vi "Puls Loop.vi"(1 "Loop ID":u16, 11 "error out":errorcluster) -> ()   [LabVIEW 2011]
uses:
  Update frequensies.ctl
  Action Analog Handler.ctl
  emi Lib/System 01/0 - General/App/Loop control 2/Private/_emi_ SMLoop start condition.vi
  emi Lib/System 01/0 - General/App/Loop control 2/Private/_emi_ SMLoop Error Check.vi
  emi Lib/Basic/0 - General/Error/emi_Is Error.vi
  emi Lib/System 01/0 - General/App/Loop control 2/Private/_emi_SMLoop Register new.vi
  emi Lib/System 01/0 - General/S&E reporting/emi_Send S&E Error message.vi
  emi Lib/Basic/0 - General/Error/emi_ Is Error state.vi
  emi Lib/System 01/0 - General/emi_Read System ID.vi
  emi Lib/System 01/0 - General/App/Loop control/Private/_emi_GFV Loop Linking.vi
  emi Lib/System 01/0 - General/App/Loop control/Private/_emi_GFV Loop Enable.vi
  emi Lib/System 01/0 - General/App/Loop control 2/Private/_emi_ SMLoop Restart.vi
  emi Lib/System 01/0 - General/App/Private/_emi_GFV App Close.vi
  emi Lib/System 01/0 - General/App/Loop control 2/Private/_emi_ SMLoop Restart Counter.vi
  emi Lib/System 01/0 - General/App/Loop control/Private/_emi_GFV Loop Running.vi
  emi Lib/System 01/0 - General/Private/_emi_GFV System ID.vi
  emi Lib/System 01/0 - General/S&E reporting/Private/_emi_S&E Q Generator.vi
  <vilib>/Utility/error.llb/Clear Errors.vi
  emi Lib/System 01/0 - General/App/Loop control/Private/_emi_GFV stop a loop so it can reset.vi
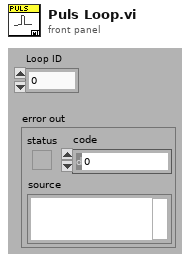
[diagram p1: front panel]
types:
  T1 = typedef "_emi_ SMLoop sates.ctl" = enum16{"Init", "Standby", "Start", "Normal Operation", "Stop", "Error Handling", "End", "Post"}
  T2 = typedef "Update frequensies.ctl" = enum16{"2 Hz", "1 Hz", "0.1 Hz"}
  T3 = typedef "Action Analog Handler.ctl" = enum16{"GET value", "GET Single Frequenzy", "GET All Values", "GET Waveform", "Get Numb Var", "SET Value", "START Buffer", "REG Variable", "BUF size(total antal sekund)", "PULS", "Get a Value at time", "Set initial waveform"}
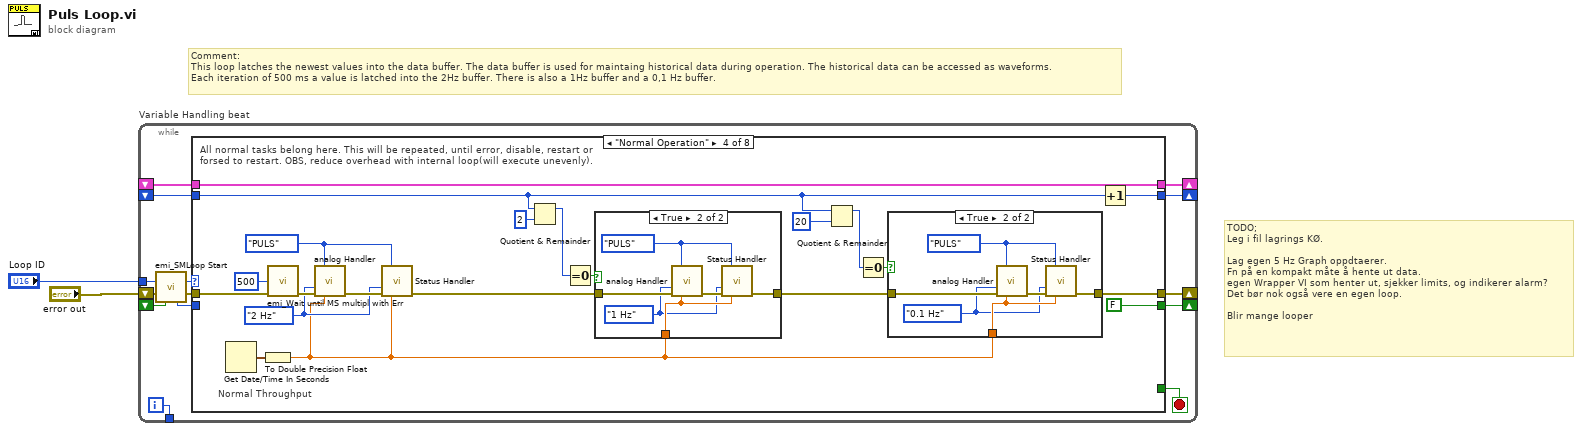
[diagram p0: block diagram]
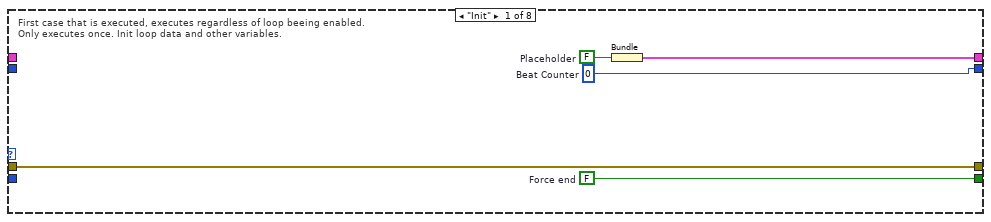
[diagram p2: hidden frame]
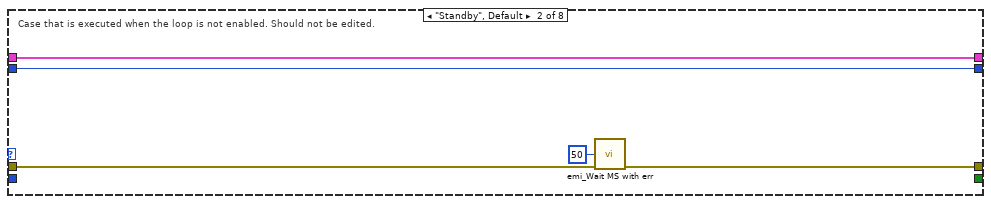
[diagram p3: hidden frame]
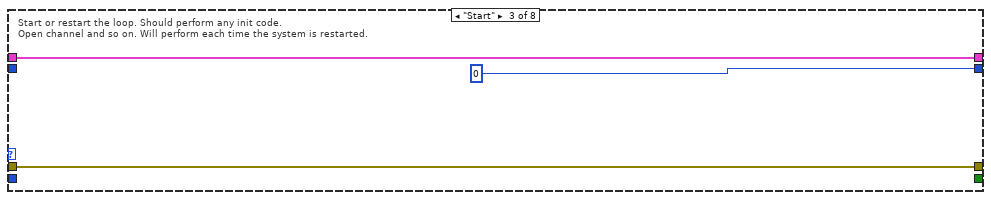
[diagram p4: hidden frame]
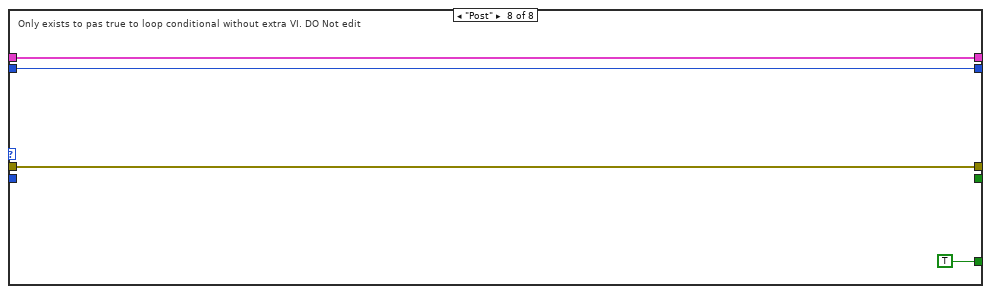
[diagram p10: hidden frame]
diagram:
  # "Comment: \nThis loop latches the newest values into the data buffer. The data buffer is used for maintaing historical data during operation. The historical data can be accessed as waveforms.\nEach iteration of 500 ms a value is latched into the 2Hz buffer. There is also a 1Hz buffer and a 0,1 Hz buffer."
  # "TODO;\nLeg i fil lagrings KØ.\n\nLag egen 5 Hz Graph oppdtaerer.\nFn på en kompakt måte å hente ut data.\negen Wrapper VI som henter ut, sjekker limits, og indikerer alarm?\nDet bør nok også vere en egen loop.\n\nBlir mange looper"
  n1 = while "Variable Handling beat" {
    shift-right: [w16] -> _
    shift-left: _ -> [w12]
    shift-right: [w14] -> _
    shift-left: "error out" -> [w10]
    tunnel: [w13] -> _
    shift-right: [w11] -> _
    shift-left: _ -> [w6]
    tunnel: "Loop ID" -> [w7]
    shift-right: [w3] -> _
    shift-left: _ -> [w4]
    i -> [w13]
    stop <- w15 stop-if-true
    n2 = call "emi_SMLoop Start.vi"("Loop ID"=w7, "error in (no error)"=w10, "Force Stop(F)"=w6) -> ("Loop command"=w8:T1, "error out"=w9:errorcluster, "Loop ID out"=w5:i32)  [unwired: 10 in]
    n3 = case shown="\"Normal Operation\"" w8 {
      tunnel: [w20 w23 w28 w48 w66 w70 w72 w76] -> w16
      tunnel: [_ _ _ _ _ _ _ TRUE] -> w15
      tunnel: w9 -> [w21 w25 w29 w50 w67 w69 w73 w77]
      tunnel: [w21 w24 w29 w49 w67 w69 w73 w77] -> w14
      tunnel: w12 -> [_ w23 w28 w48 w66 w70 w72 w76]
      tunnel: [w18 _ _ FALSE ("Force End") _ _ _ _] -> w11
      tunnel: w5 -> [_ _ _ _ _ _ _ _]
      tunnel: w4 -> [_ w22 _ w46 w65 w68 w71 w74]
      tunnel: [w17 w22 0 ("Beat Counter") w45 w65 w68 w71 w74] -> w3
      frame "Init" {
        w17 = 0  # Beat Counter
        w18 = FALSE  # Force end
        w19 = FALSE  # Placeholder
        # "First case that is executed, executes regardless of loop beeing enabled.\nOnly executes once. Init loop data and other variables."
        n4 = Bundle("Placeholder"=w19) -> (w20:cluster{"Placeholder":bool})  [unwired: 1 in]
      }
      frame "Standby", Default {
        # "Case that is executed when the loop is not enabled. Should not be edited."
        n5 = call "emi_Wait MS with err.vi"("milliseconds to wait(0)"=u32 50, "error in (no error)"=w25) -> ("error out"=w24:errorcluster)  [unwired: 13 in]
      }
      frame "Start" {
        # "Start or restart the loop. Should perform any init code. \nOpen channel and so on. Will perform each time the system is restarted."
      }
      frame "Normal Operation" {
        w31 = Update_frequensies."2 Hz" ("Upd freq")
        w32 = Action_Analog_Handler."PULS" ("Action(GET)")
        # "Normal Throughput"
        # "All normal tasks belong here. This will be repeated, until error, disable, restart or\nforsed to restart. OBS, reduce overhead with internal loop(will execute unevenly)."
        n6 = Get Date/Time In Seconds() -> (seconds since 1Jan1904=w35:timestamp)
        n7 = To Double Precision Float(number=w35) -> (double precision float=w30:dbl)
        n8 = call "emi_Wait until MS multipl with Err.vi"("millisecond multiple(0)"=u32 500, "error in (no error)"=w50) -> ("error out"=w43:errorcluster)  [unwired: 13 in]
        n9 = call "analog Handler.vi"("Action"=w32, "Upd freq"=w31, "error in (no error)"=w43, "Start tid / buf size"=w30) -> ("error out"=w34:errorcluster)  [unwired: 6 in, 5 out]
        n10 = call "Status Handler.vi"("Action"=w32, "Upd freq"=w31, "error in (no error)"=w34, "Start tid(buff size"=w30) -> ("error out"=w33:errorcluster)  [unwired: 7 in, 4 out]
        n11 = Quotient & Remainder(x=w46, y=2) -> (x-y*floor(x/y)=w40:i32)  [unwired: 1 out]
        n12 = Equal To 0?(x=w40) -> (x = 0?=w38:bool)
        n13 = case shown="True" w38 {
          tunnel: w33 -> [w58 w64]
          tunnel: [w58 w63] -> w36
          tunnel: w30 -> [_ w61]
          frame False {
          }
          frame True {
            w60 = Update_frequensies."1 Hz" ("Upd freq")
            w59 = Action_Analog_Handler."PULS" ("Action(GET)")
            n14 = call "analog Handler.vi"("Action"=w59, "Upd freq"=w60, "error in (no error)"=w64, "Start tid / buf size"=w61) -> ("error out"=w62:errorcluster)  [unwired: 6 in, 5 out]
            n15 = call "Status Handler.vi"("Action"=w59, "Upd freq"=w60, "error in (no error)"=w62, "Start tid(buff size"=w61) -> ("error out"=w63:errorcluster)  [unwired: 7 in, 4 out]
          }
        }
        n16 = Quotient & Remainder(x=w46, y=20) -> (x-y*floor(x/y)=w39:i32)  [unwired: 1 out]
        n17 = Equal To 0?(x=w39) -> (x = 0?=w37:bool)
        n18 = case shown="True" w37 {
          tunnel: w36 -> [w51 w57]
          tunnel: [w51 w55] -> w49
          tunnel: w30 -> [_ w54]
          frame False {
          }
          frame True {
            w53 = Update_frequensies."0.1 Hz" ("Upd freq")
            w52 = Action_Analog_Handler."PULS" ("Action(GET)")
            n19 = call "analog Handler.vi"("Action"=w52, "Upd freq"=w53, "error in (no error)"=w57, "Start tid / buf size"=w54) -> ("error out"=w56:errorcluster)  [unwired: 6 in, 5 out]
            n20 = call "Status Handler.vi"("Action"=w52, "Upd freq"=w53, "error in (no error)"=w56, "Start tid(buff size"=w54) -> ("error out"=w55:errorcluster)  [unwired: 7 in, 4 out]
          }
        }
        n21 = Increment(x=w46) -> (x+1=w45:i32)
      }
      frame "Stop" {
        # "Stop the loop. May be restarted later. Close interfaces and the like"
      }
      frame "Error Handling" {
        # "Loop automaticaly returns here after error is found. If error is cleared, \nLoop wil continue as normal(if was operative when error."
      }
      frame "End" {
        # "Only executes at application end has. Should performa any action the loop \nneeds to finnish. Executes only once."
      }
      frame "Post" {
        # "Only exists to pas true to loop conditional without extra VI. DO Not edit"
      }
    }
  }
